vi "Calculate Desired States.vi"(8 "error in (no error)":errorcluster, 10 "Vessel In":refnum<class "Vessel.lvclass">, 11 "CJ switcher in":refnum<class "CJ switcher.lvclass">) -> (0 "error out":errorcluster, 2 "Vessel Out":refnum<class "Vessel.lvclass">, 3 "CJ switcher out":refnum<class "CJ switcher.lvclass">)   [LabVIEW 2014, in "Guidance Library.lvlib" / "CJ switcher.lvclass"]
uses:
  CJ switcher.lvclass
  ROV/Vessel.lvclass
  Library/Helping Routines/get_set_point_vec (SubVI).vi
  <vilib>/imath/engines/lvmath2/RunTimeEngine/Managers/WorkSpace/UID Generator.vi
  <vilib>/imath/engines/lvmath2/RunTimeEngine/RunTimeType/NIMS_RunTimeType_From StrictType (excl LVString).vi
  <instcachedir>/0/NIMS_RunTimeType_From StrictType (excl LVString)_15A5391EEA9C4AACB9955AC755B83D29.lvgen/NIMS_RunTimeType_From StrictType (excl LVString)_15A5391EEA9C4AACB9955AC755B83D29_000.vi
  <vilib>/imath/engines/lvmath2/RunTimeEngine/LocalVariableDefStatement/MC_LocalVariableDefStatement_Display.vi
  <vilib>/imath/engines/lvmath2/RunTimeEngine/BuiltInFunctions/size/NIMS_[I32,I32]=size(GM).vi
  <instcachedir>/0/NIMS_[I32,I32]=size(GM)_B0A6EC1255BB4C8AB801FE6F734128D9.lvgen/NIMS_[I32,I32]=size(GM)_B0A6EC1255BB4C8AB801FE6F734128D9_000.vi
  <vilib>/imath/engines/lvmath2/RunTimeEngine/IndexRead/NIMS V(R2).vi
  <instcachedir>/0/NIMS V(R2)_C76619605A0E4E9F8B2FA9389712AC47.lvgen/NIMS V(R2)_C76619605A0E4E9F8B2FA9389712AC47_000.vi
  <vilib>/imath/engines/lvmath2/RunTimeEngine/IndexRead/NIMS M(S,R2).vi
  <instcachedir>/0/NIMS M(S,R2)_45730E4D0DB74D118F715F4F99DCE4D7.lvgen/NIMS M(S,R2)_45730E4D0DB74D118F715F4F99DCE4D7_000.vi
  <vilib>/imath/engines/lvmath2/RunTimeEngine/ArithmeticOperatorToken/NIMS_ArithmeticOperator_multmx(M,CV)-internal.vi
  <instcachedir>/0/NIMS_ArithmeticOperator_multmx(M,CV)-internal_25C7CE5937BA4322B5BE2717374345EA.lvgen/NIMS_ArithmeticOperator_multmx(M,CV)-internal_25C7CE5937BA4322B5BE2717374345EA_001.vi
  <vilib>/imath/engines/lvmath2/RunTimeEngine/ErrorHandling/NIMS_Create Error From Enums.vi
  <vilib>/imathl/engines/lvmath/Functions/Error Handling/Create Error.vi
  <vilib>/imath/engines/lvmath2/RunTimeEngine/IndexRead/NIMS V(S).vi
  <instcachedir>/0/NIMS V(S)_0488751826AF41519A22953C041130DC.lvgen/NIMS V(S)_0488751826AF41519A22953C041130DC_000.vi
  <vilib>/imath/engines/lvmath2/RunTimeEngine/BuiltInFunctions/atan2/NIMS_atan2.vi
  <instcachedir>/0/NIMS_atan2_A91AA4A7D42247EDBE8F76DB99AF04A4.lvgen/NIMS_atan2_A91AA4A7D42247EDBE8F76DB99AF04A4_000.vi
  <vilib>/imath/engines/lvmath2/RunTimeEngine/IndexReplace/NIMS M(S,R2)=V.vi
  <instcachedir>/0/NIMS M(S,R2)=V_74719D1886FD41299CC34F2C1799E6B7.lvgen/NIMS M(S,R2)=V_74719D1886FD41299CC34F2C1799E6B7_000.vi
  <vilib>/imath/engines/lvmath2/RunTimeEngine/BuiltInFunctions/abs/NIMS_abs(signed).vi
  <instcachedir>/0/NIMS_abs(signed)_C4FCB8E6058B49B797C7C8D53CA5F6EC.lvgen/NIMS_abs(signed)_C4FCB8E6058B49B797C7C8D53CA5F6EC_000.vi
  <vilib>/imath/engines/lvmath2/RunTimeEngine/Managers/SymbolTable/Clear UID.vi
  <vilib>/imath/engines/lvmath2/RunTimeEngine/NodeEndStatement/NIMS_NodeEndStatement_Output.vi
  <instcachedir>/0/NIMS_NodeEndStatement_Output_53EC0D466D134D7ABD903AC30B43404B.lvgen/NIMS_NodeEndStatement_Output_53EC0D466D134D7ABD903AC30B43404B_005.vi
  <instcachedir>/0/NIMS_NodeEndStatement_Output_53EC0D466D134D7ABD903AC30B43404B.lvgen/NIMS_NodeEndStatement_Output_53EC0D466D134D7ABD903AC30B43404B_012.vi
  <instcachedir>/0/NIMS_NodeEndStatement_Output_53EC0D466D134D7ABD903AC30B43404B.lvgen/NIMS_NodeEndStatement_Output_53EC0D466D134D7ABD903AC30B43404B_001.vi
  <instcachedir>/0/NIMS_NodeEndStatement_Output_53EC0D466D134D7ABD903AC30B43404B.lvgen/NIMS_NodeEndStatement_Output_53EC0D466D134D7ABD903AC30B43404B_011.vi
  <vilib>/imath/engines/lvmath2/RunTimeEngine/ErrorHandling/NIMS_Finalize Error.vi
  Constant Jerk Guidance/Constant Jerk Guidance.lvclass
  Supervisor/Supervisor.lvclass
  <vilib>/imath/engines/lvmath2/RunTimeEngine/Managers/SymbolTable/NIMS_WorkSpace.lvlib
panel:
  out "dove":i32
  out "eps_t":dbl[](array[numeric])
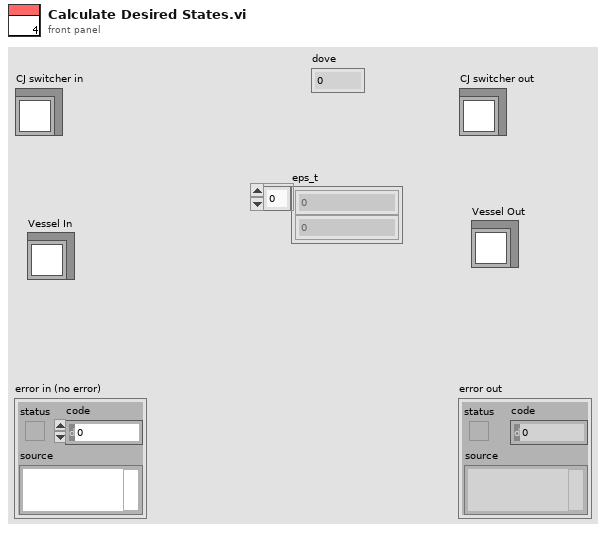
[diagram p1: front panel]
types:
  T1 = cluster{"Performance Behavior":cluster{"% Velocity max lin to exp":dbl, "% Velocity zero lin to exp":dbl, "% Total dist at max velocity":dbl, "Max angular velocity":dbl, "Time to max linear velocity":dbl, "Min dist at max velocity":dbl, "Max linear velocity":dbl, "Time to max angular velocity":dbl}, "Table of WP":dbl[][], "Tracking Options":cluster{"Superior Bound":dbl, "Inferior Bound":dbl, "Duration No operation period between motions":dbl, "Tolerance of initial angle":dbl, "Distance to activation waiting function":dbl, "Distance to deactivation waiting function":dbl, "(2) Fixed Heading":dbl, "(3) PoI N":dbl, "(3) PoI E":dbl}, "Start":bool, "Use Position":bool, "Heading Mode":u16, "Pause":bool, "Abort":bool}
  T2 = cluster{"javp":dbl[], " javr":dbl[], "Break":bool, "arrived":bool, "arrived yaw":bool}
  T3 = cluster{"Measured":cluster{"Eta":dbl[], "Nu":dbl[], "Eta Dot":dbl[], "Nu Dot":dbl[]}, "Estimated":cluster{"Eta":dbl[], "Nu":dbl[], "Eta Dot":dbl[], "Nu Dot":dbl[]}, "Desired":cluster{"Eta":dbl[], "Nu":dbl[], "Eta Dot":dbl[], "Nu Dot":dbl[]}, "Previous Desired":cluster{"Eta":dbl[], "Nu":dbl[], "Eta Dot":dbl[], "Nu Dot":dbl[]}, "tau":dbl[], "Altitude":cluster{"Measured":dbl, "Estimated":dbl, "Desired":dbl, "Previous Desired":dbl, "Approximated":dbl, "grad F":dbl[]}, "rpm":dbl[], "Attitude":cluster{"Theta Measured":dbl[], "Theta Estimated":dbl[], "Omega Measured":dbl[], "Omega Estimated":dbl[], "Gyro Bias":dbl[]}}
  T4 = cluster{"Set Origin":bool, "New WP":bool, "Types of Change":enum16{"Current NED", "Change NED"}, "Make Change":bool, "Optimal Heading":bool, "New SetPoint":cluster{"North":dbl, "East":dbl, "Depth":dbl, "Heading":dbl}, "Update Reference":cluster{"Mode Change":bool, "Current Position":dbl[]}, "Go":bool, "Go heading":bool}
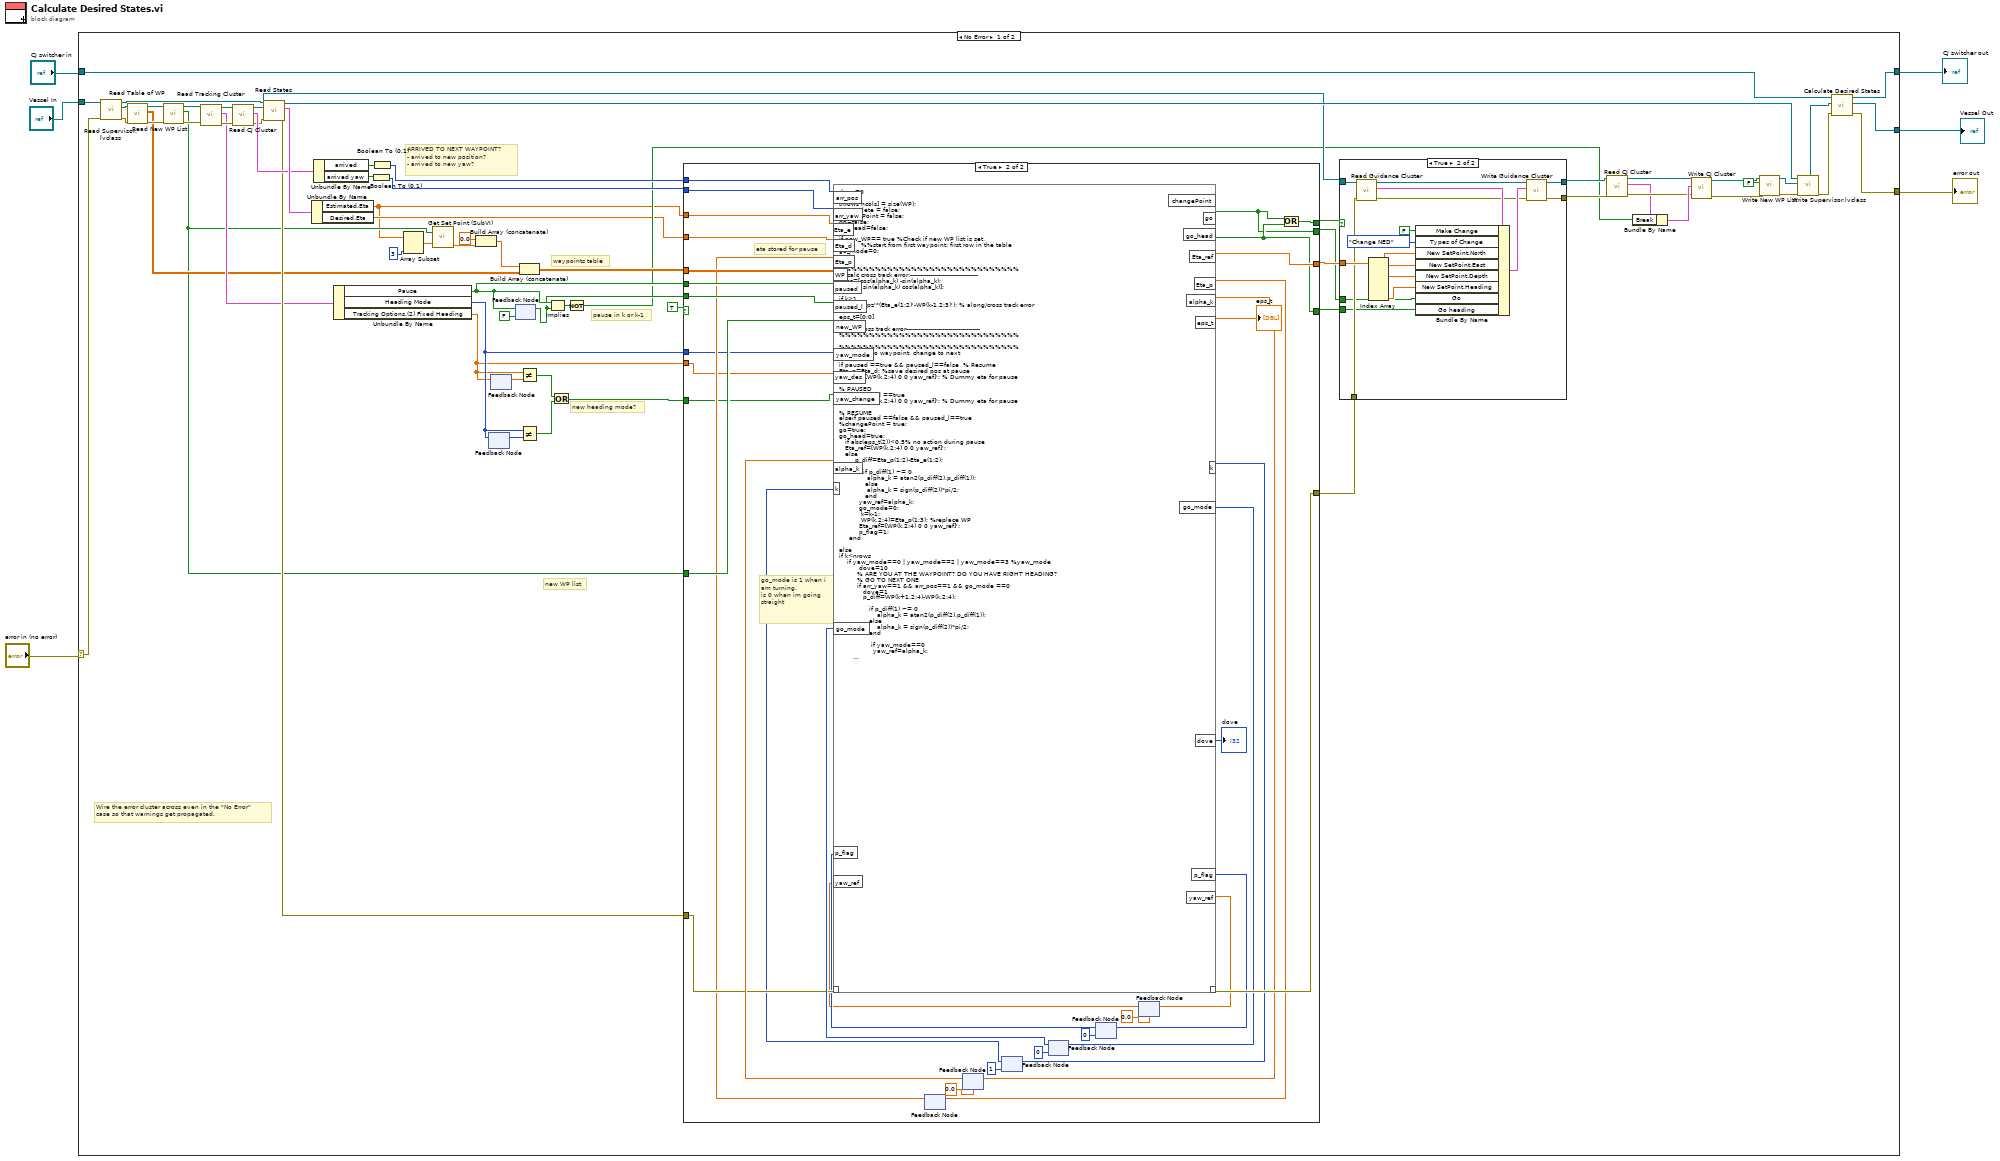
[diagram p0: block diagram]
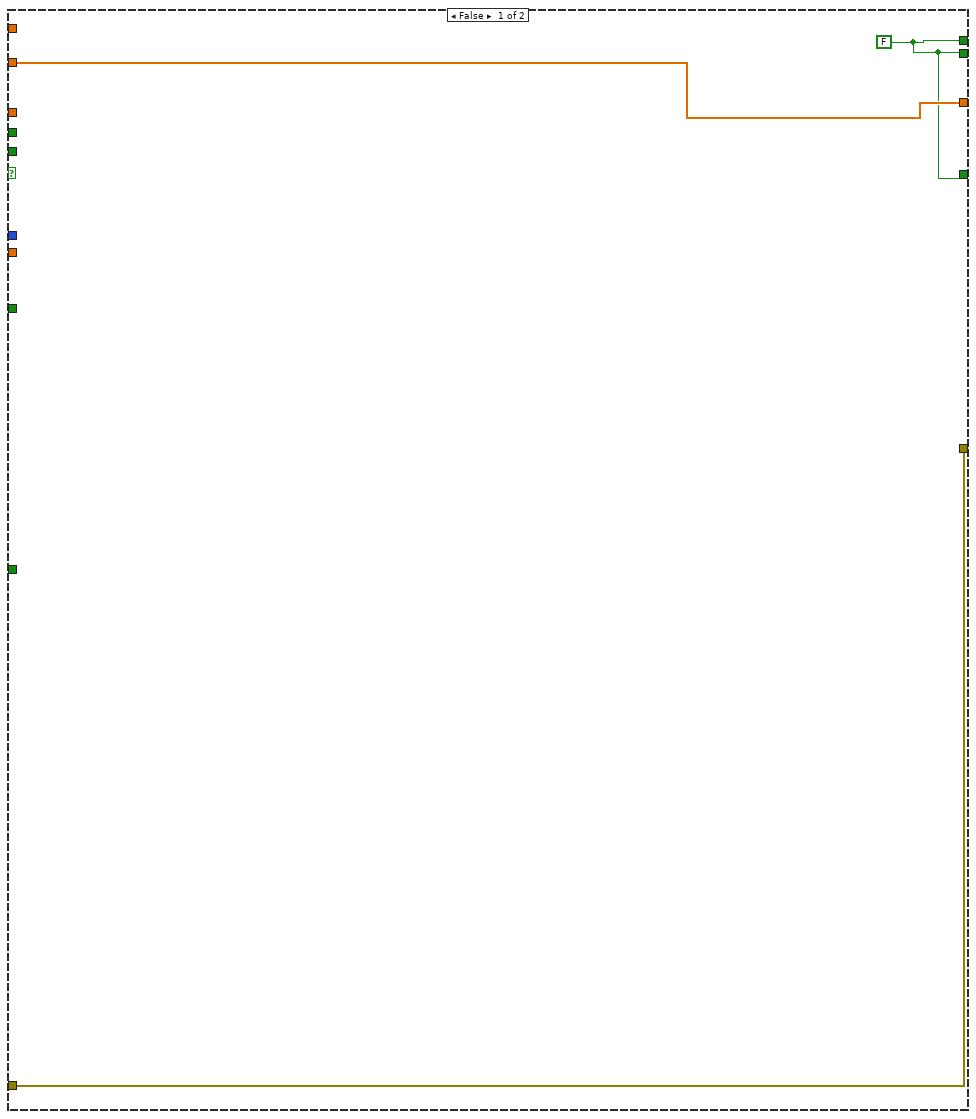
[diagram p3: hidden frame]
diagram:
  n1 = case shown="No Error" "error in (no error)" {
    selector: "error in (no error)" -> [w62 w1927]
    tunnel: [w58 w1927] -> w5
    tunnel: [w72 w1926] -> w3
    tunnel: "CJ switcher in" -> [w73 w1926]
    tunnel: "Vessel In" -> [w63 w1925]
    tunnel: [w71 w1925] -> w1
    frame No Error {
      # "new WP list"
      # "pause in k or k-1"
      # "new heading mode?"
      # "waypoints table"
      # "ARRIVED TO NEXT WAYPOINT?\n- arrived to new position?\n- arrived to new yaw?"
      # "Wire the error cluster across even in the \"No Error\"\ncase so that warnings get propagated."
      n2 = call "Read Supervisor.lvclass.vi"("error in (no error)"=w62, "Vessel in"=w63) -> ("error out"=w61:errorcluster, "Supervisor.lvclass"=w69:refnum<class "Supervisor.lvclass">, "Vessel out"=w66:refnum<class "Vessel.lvclass">)  [unwired: 7 in]
      n3 = call-dynamic "Read Table of WP.vi"("error in (no error)"=w61, "Supervisor in"=w69) -> ("error out"=w50:errorcluster, "Table of WP"=w38:dbl[][], "Supervisor out"=w64:refnum<class "Supervisor.lvclass">)  [unwired: 7 in]
      n4 = call-dynamic "Read New WP List.vi"("error in (no error)"=w50, "Supervisor in"=w64) -> ("error out"=w41:errorcluster, "New WP List"=w34:bool, "Supervisor out"=w44:refnum<class "Supervisor.lvclass">)  [unwired: 7 in]
      n5 = call-dynamic "Read Tracking Cluster.vi"("error in (no error)"=w41, "Supervisor in"=w44) -> ("error out"=w43:errorcluster, "Tracking Cluster"=w40:T1, "Supervisor out"=w42:refnum<class "Supervisor.lvclass">)  [unwired: 7 in]
      n6 = call-dynamic "Read CJ Cluster.vi"("error in (no error)"=w43, "Supervisor in"=w42) -> ("error out"=w49:errorcluster, "CJ Cluster"=w55:T2, "Supervisor out"=w56:refnum<class "Supervisor.lvclass">)  [unwired: 7 in]
      n7 = call-dynamic "Read States.vi"("error in (no error)"=w49, "Vessel in"=w66) -> ("error out"=w48:errorcluster, "States"=w70:T3, "Vessel out"=w65:refnum<class "Vessel.lvclass">)  [unwired: 7 in]
      n8 = Unbundle By Name(w70) -> ("Estimated.Eta"=w16:dbl[], "Desired.Eta"=w17:dbl[])
      n9 = Unbundle By Name(w55) -> ("arrived"=w54:bool, "arrived yaw"=w53:bool)
      n10 = Unbundle By Name(w40) -> ("Pause"=w21:bool, "Heading Mode"=w8:u16, "Tracking Options.(2) Fixed Heading"=w7:dbl)
      n11 = Boolean To (0,1)(Boolean=w53) -> (0, 1=w51:i16)
      n12 = Boolean To (0,1)(Boolean=w54) -> (0, 1=w52:i16)
      n13 = Array Subset(array=w16, length=3) -> (w35:dbl[])  [unwired: 1 in]
      n14 = call-poly "Get Set Point (SubVI).vi"("Set point in"=w35, "auto set  in"=w34) -> ("Set point"=w32:dbl[])  [unwired: 1 out]
      n15 = Build Array (concatenate)(0.0 ("element"), w32) -> (w31:dbl[])
      n16 = feedback #1() -> (w12:u16)  [unwired: 1 in]
      n17 = feedback-in #1(w8) -> ()
      n18 = feedback-in #2(w7) -> ()
      n19 = feedback #2() -> (w15:dbl)  [unwired: 1 in]
      n20 = feedback #3(FALSE ("paused")) -> (w20:bool)
      n21 = feedback-in #3(w21) -> ()
      n22 = Build Array (concatenate)(w31, w38) -> (w36:dbl[][])
      n23 = Not Equal?(x=w7, y=w15) -> (x != y?=w10:bool)
      n24 = Not Equal?(x=w8, y=w12) -> (x != y?=w11:bool)
      n25 = Implies(1:w20, 2:w21) -> (0:w19:bool)
      n26 = Or(x=w10, y=w11) -> (x .or. y?=w9:bool)
      n27 = Not(x=w19) -> (.not. x?=w18:bool)
      n28 = case shown="True" TRUE {
        tunnel: w36 -> [_ w131]
        tunnel: [w94 w123] -> w67
        tunnel: [w95 w127] -> w60
        tunnel: w17 -> [w94 w129]
        tunnel: [w93 w100] -> w68
        tunnel: w34 -> [_ w116]
        tunnel: w48 -> [w95 w126]
        tunnel: w52 -> [_ w125]
        tunnel: w51 -> [_ w124]
        tunnel: w21 -> [_ w120]
        tunnel: w20 -> [_ w119]
        tunnel: w16 -> [_ w113]
        tunnel: w8 -> [_ w105]
        tunnel: w7 -> [_ w104]
        tunnel: w9 -> [_ w103]
        tunnel: [w93 w101] -> w14
        tunnel: [w93 w102] -> w13
        frame False {
          w93 = FALSE ("changePoint")
        }
        frame True {
          # "go_mode is 1 when i am turning.\nis 0 when im going straight"
          # "eta stored for pause"
          n29 = feedback #4() -> (w114:dbl[])  [unwired: 1 in]
          n30 = feedback #5(0.0 ("WP_Index")) -> (w128:dbl)
          n31 = feedback #6(1 ("k")) -> (w122:i32)
          n32 = feedback #7(0 ("go_mode")) -> (w130:i32)
          n33 = feedback #8(0 ("p_flag")) -> (w106:i32)
          n34 = feedback #9(0.0 ("WP_Index")) -> (w97:dbl)
          n35 = mathscript code="dove=0\n\n[nrows ncols] = size(WP);\n%complete = false;\nchangePoint = false;\ngo=false;\ngo_head=false;\n\nif new_WP== true %Check if new WP list is set.\nk=1;    %%start from first waypoint: first row in the table\ngo_mode=0;\nend\n\n%%%%%%%%%%%%%%%%%%%%%%%%%%%%%%\n% calc cross track error:----------------------------------\nR_pz=[cos(alpha_k) -sin(alpha_k);\n            sin(alpha_k) cos(alpha_k)];\n\nif k>1\neps_t=R_pz'*(Eta_e(1:2)'-WP(k-1,2:3)'); % along/cross track error\nelse\neps_t=[0;0]\nend\n%end cross track error-------------------------------------\n%%%%%%%%%%%%%%%%%%%%%%%%%%%%%%\n\n%%%%%%%%%%%%%%%%%%%%%%%%%%%%%%\n% Is close to waypoint, change to next\n\nif paused ==true && paused_l==false  % Resume\nEta_p=Eta_d; %save desired pos at pause\nEta_ref=[WP(k,2:4) 0 0 yaw_ref]'; % Dummy eta for pause\n\n% PAUSED\nelseif paused ==true  \nEta_ref=[WP(k,2:4) 0 0 yaw_ref]'; % Dummy eta for pause\n\n% RESUME\nelseif paused ==false && paused_l==true  \n%changePoint = true;\ngo=true;\ngo_head=true;\n   if abs(eps_t(2))<0.5% no action during pause\n   Eta_ref=[WP(k,2:4) 0 0 yaw_ref]';\n   else\n        p_diff=Eta_p(1:2)-Eta_e(1:2);\n\n            if p_diff(1) ~= 0\n              alpha_k = atan2(p_diff(2),p_diff(1));\n             else\n              alpha_k = sign(p_diff(2))*pi/2;\n             end\n          yaw_ref=alpha_k;\n          go_mode=0;\n           k=k-1;\n           WP(k,2:4)=Eta_p(1:3); %replace WP\n          Eta_ref=[WP(k,2:4) 0 0 yaw_ref]';\n          p_flag=1;\n     end\n\nelse\nif k<nrows\n    if yaw_mode==0 | yaw_mode==2 | yaw_mode==3 %yaw_mode\n          dove=10\n         % ARE YOU AT THE WAYPOINT? DO YOU HAVE RIGHT HEADING?\n         % GO TO NEXT ONE\n         if arr_yaw==1 && arr_pos==1 && go_mode ==0\n            dove=1\n            p_diff=WP(k+1,2:4)-WP(k,2:4);\n\n               if p_diff(1) ~= 0\n                   alpha_k = atan2(p_diff(2),p_diff(1));\n               else\n                   alpha_k = sign(p_diff(2))*pi/2;\n               end\n\n                if yaw_mode==0\n                 yaw_ref=alpha_k;\n                elseif yaw_mode==2\n                 yaw_ref=alpha_k+pi/2;\n                elseif yaw_mode==3\n                 yaw_ref=alpha_k-pi/2;\n                end\n             %changePoint = true;\n             go_head=true;\n             go_mode=1;\n             arr_yaw=0;  % FIRST CHANGE HEADING: not arrived to new heading\n\n                 if p_flag==1 % go to pause point at resume\n                       WP(k,2:4)=Eta_p(1:3); %replace WP\n                       p_flag=0;\n                 end\n\n         elseif arr_yaw==1 && go_mode ==1\n            dove=2\n             %changePoint = true;\n             go=true;\n              k=k+1;\n             go_mode=0;\n          elseif yaw_change==true\n          dove=3\n                 if yaw_mode==0\n                 yaw_ref=alpha_k;\n                elseif yaw_mode==2\n                 yaw_ref=alpha_k+pi/2;\n                elseif yaw_mode==3\n                 yaw_ref=alpha_k-pi/2;\n                end\n                 go_head=true;\n          else\n% hva da?\n%run=1;\n          end\n    else %yaw mode\n          if arr_pos==1\n             p_diff=WP(k+1,2:4)-WP(k,2:4);\n               if p_diff(1) ~= 0\n                   alpha_k = atan2(p_diff(2),p_diff(1));\n               else\n                   alpha_k = sign(p_diff(2))*pi/2;\n               end\n             k=k+1;\n             go=true;\n          end\n          if yaw_change==true\n           yaw_ref=yaw_des;\n           go_head=true;\n          end\n    end %yaw_mode\n\n        Eta_ref=[WP(k,2:4) 0 0 yaw_ref]';\n\n   else %norows\n       if yaw_mode==0 | yaw_mode==2 | yaw_mode==3 %yaw mode\n           if yaw_change==true\n                if yaw_mode==0\n                 yaw_ref=alpha_k;\n                elseif yaw_mode==2\n                 yaw_ref=alpha_k+pi/2;\n                elseif yaw_mode==3\n                 yaw_ref=alpha_k-pi/2;\n                end\n           go_head=true;\n          end\n     else %yaw_mode\n           if yaw_change==true\n           yaw_ref=yaw_des;\n           go_head=true;\n          end\n     end\n        Eta_ref=[WP(nrows,2:4) 0 0 yaw_ref]';\n   end %norows\nend %pause"("??"=w126, "WP"=w131, "k"=w122, "Eta_d"=w129, "go_mode"=w130, "paused"=w120, "alpha_k"=w128, "arr_pos"=w125, "arr_yaw"=w124, "paused_l"=w119, "new_WP"=w116, "Eta_p"=w114, "Eta_e"=w113, "p_flag"=w106, "yaw_mode"=w105, "yaw_des"=w104, "yaw_change"=w103, "yaw_ref"=w97) -> ("??"=w127:errorcluster, "Eta_ref"=w123:dbl[], "Eta_p"=w115:dbl[], "alpha_k"=w112:dbl, "eps_t"=→"eps_t":dbl[], "k"=w110:i32, "go_mode"=w109:i32, "p_flag"=w108:i32, "go"=w101:bool, "go_head"=w102:bool, "yaw_ref"=w98:dbl, "dove"=→"dove":i32)  [unwired: 1 out]
          n36 = feedback-in #4(w115) -> ()
          n37 = feedback-in #5(w112) -> ()
          n38 = feedback-in #6(w110) -> ()
          n39 = feedback-in #7(w109) -> ()
          n40 = feedback-in #8(w108) -> ()
          n41 = feedback-in #9(w98) -> ()
          n42 = Or(x=w101, y=w102) -> (x .or. y?=w100:bool)
        }
      }
      n43 = case shown="True" w68 {
        tunnel: w56 -> [w75 w92]
        tunnel: w67 -> [_ w89]
        tunnel: [w75 w80] -> w26
        tunnel: w60 -> [w74 w82]
        tunnel: [w74 w79] -> w25
        tunnel: w14 -> [_ w78]
        tunnel: w13 -> [_ w77]
        frame False {
        }
        frame True {
          n44 = call-dynamic "Read Guidance Cluster.vi"("error in (no error)"=w82, "Supervisor in"=w92) -> ("error out"=w81:errorcluster, "Guidance Cluster"=w91:T4, "Supervisor out"=w83:refnum<class "Supervisor.lvclass">)  [unwired: 7 in]
          n45 = Index Array(array=w89) -> (element #1=w88:dbl, element #2=w87:dbl, element #3=w86:dbl, element #6=w85:dbl)  [unwired: 6 in, 2 out]
          n46 = Bundle By Name(cluster=w91, "Make Change"=FALSE, "Types of Change"=enum16{"Current NED", "Change NED"}."Change NED", "New SetPoint.North"=w88, "New SetPoint.East"=w87, "New SetPoint.Depth"=w86, "New SetPoint.Heading"=w85, "Go"=w78, "Go heading"=w77) -> (w84:T4)
          n47 = call-dynamic "Write Guidance Cluster.vi"("error in (no error)"=w81, "Guidance Cluster"=w84, "Supervisor in"=w83) -> ("error out"=w79:errorcluster, "Supervisor out"=w80:refnum<class "Supervisor.lvclass">)  [unwired: 7 in]
        }
      }
      n48 = call-dynamic "Read CJ Cluster.vi"("error in (no error)"=w25, "Supervisor in"=w26) -> ("error out"=w29:errorcluster, "CJ Cluster"=w27:T2, "Supervisor out"=w28:refnum<class "Supervisor.lvclass">)  [unwired: 7 in]
      n49 = Bundle By Name(cluster=w27, "Break"=w18) -> (w30:T2)
      n50 = call-dynamic "Write CJ Cluster.vi"("error in (no error)"=w29, "CJ Cluster"=w30, "Supervisor in"=w28) -> ("error out"=w23:errorcluster, "Supervisor out"=w24:refnum<class "Supervisor.lvclass">)  [unwired: 7 in]
      n51 = call-dynamic "Write New WP List.vi"("error in (no error)"=w23, "New WP List"=FALSE, "Supervisor in"=w24) -> ("error out"=w47:errorcluster, "Supervisor out"=w46:refnum<class "Supervisor.lvclass">)  [unwired: 7 in]
      n52 = call "Write Supervisor.lvclass.vi"("error in (no error)"=w47, "Supervisor.lvclass"=w46, "Vessel in"=w65) -> ("error out"=w59:errorcluster, "Vessel out"=w57:refnum<class "Vessel.lvclass">)  [unwired: 7 in]
      n53 = call-parent "Calculate Desired States.vi"("error in (no error)"=w59, "Vessel In"=w57, "CJ Constant Jerk Guidance in"=w73) -> ("error out"=w58:errorcluster, "Vessel Out"=w71:refnum<class "Vessel.lvclass">, "CJ Constant Jerk Guidance out"=w72:refnum<class "CJ switcher.lvclass">)  [unwired: 6 in]
    }
    frame Error {
    }
  }
  "error out" <- w5
  "CJ switcher out" <- w3
  "Vessel Out" <- w1
